vi "Instr_InitObject.vi"(8 "error in (no error)":errorcluster, 9 "Instrument Configuration":variant, 10 "Instrument address":refnum<visa-resource-name>, 11 "KE6517 in":refnum<class "KE6517.lvclass">) -> (0 "error out":errorcluster, 3 "KE6517 out":refnum<class "KE6517.lvclass">)   [LabVIEW 2018, in "KE6517.lvclass"]
uses:
  KE6517.lvclass
  InstrumentSetup.vi
  KE6517_CommandsGlobal.vi
  SupplyControl.lvclass
  InstrControl.lvclass
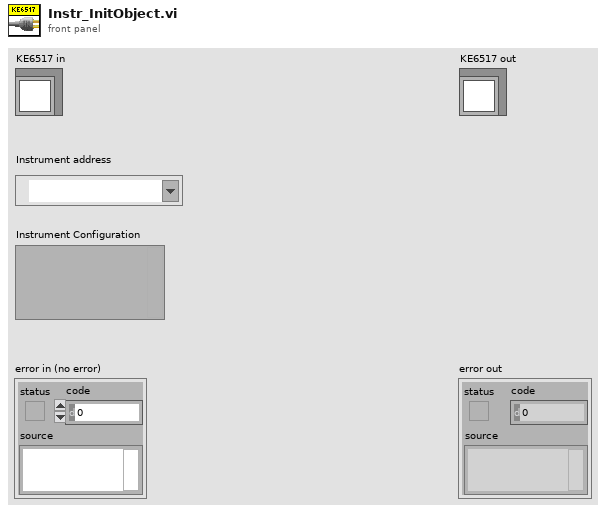
[diagram p1: front panel]
types:
  T1 = cluster{"Compliance [A]":sgl, "Voltage range (source)":enum16{"Auto", "200 V", "500 V", "1500 V", "3000 V"}, "Current range (measure)":enum16{"Auto", "1 nA", "10 nA", "100 nA", "1 uA", "10 uA", "100 uA", "1 mA", "2 mA", "20 mA", "120 mA"}, "KE2657A":refnum<class "KE2657A.lvclass">}
  T2 = cluster{"Instrument name":string, "Command \"Reset\"":string, "Command \"Initialise\"":string, "Command \"Arm\"":string, "Command \"SetVolts\"":string, "Command \"Compliance?\"":string, "Command \"Standby\"":string, "Command \"Read Current\"":string}
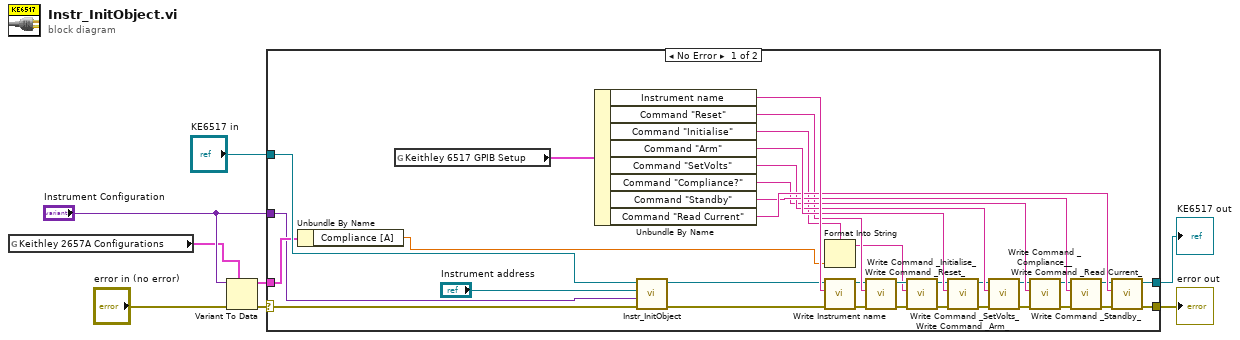
[diagram p0: block diagram]
diagram:
  n1 = global read "InstrumentSetup.vi" "Keithley 2657A Configurations"() -> (w2:T1)
  n2 = Variant To Data(error in="error in (no error)", type=w2, Variant="Instrument Configuration") -> (data=w1:T1, error out=w4:errorcluster)
  n3 = case shown="No Error" w4 {
    selector: w4 -> [w12 w44]
    tunnel: [w22 w44] -> w6
    tunnel: [w23 w43] -> w7
    tunnel: "KE6517 in" -> [w15 w43]
    tunnel: w1 -> [w10 _]
    tunnel: "Instrument Configuration" -> [w9 _]
    frame No Error {
      n4 = Unbundle By Name(w10) -> ("Compliance [A]"=w21:sgl)
      n5 = global read "KE6517_CommandsGlobal.vi" "Keithley 6517 GPIB Setup"() -> (w18:T2)
      n6 = Unbundle By Name(w18) -> ("Instrument name"=w42:string, "Command \"Reset\""=w36:string, "Command \"Initialise\""=w20:string, "Command \"Arm\""=w41:string, "Command \"SetVolts\""=w38:string, "Command \"Compliance?\""=w37:string, "Command \"Standby\""=w39:string, "Command \"Read Current\""=w40:string)
      n7 = call-parent "Instr_InitObject.vi"("error in (no error)"=w12, "Instrument Configuration"=w9, "Instrument address"="Instrument address", "SupplyControl in"=w15) -> ("error out"=w11:errorcluster, "SupplyControl out"=w14:refnum<class "KE6517.lvclass">)  [unwired: 6 in]
      n8 = Format Into String(format string=w20, w21) -> (resulting string=w19:string)  [unwired: 2 in, 1 out]
      n9 = call-dynamic "Write Instrument name.vi"("error in (no error)"=w11, "Instrument name"=w42, "InstControl in"=w14) -> ("error out"=w16:errorcluster, "InstControl out"=w17:refnum<class "KE6517.lvclass">)  [unwired: 7 in]
      n10 = call-dynamic "Write Command _Reset_.vi"("error in (no error)"=w16, "Command \"Reset\""=w36, "SupplyControl in"=w17) -> ("error out"=w29:errorcluster, "SupplyControl out"=w35:refnum<class "KE6517.lvclass">)  [unwired: 7 in]
      n11 = call-dynamic "Write Command _Initialise_.vi"("error in (no error)"=w29, "Command \"Initialise\""=w19, "SupplyControl in"=w35) -> ("error out"=w28:errorcluster, "SupplyControl out"=w34:refnum<class "KE6517.lvclass">)  [unwired: 7 in]
      n12 = call-dynamic "Write Command _Arm_.vi"("error in (no error)"=w28, "Command \"Arm\""=w41, "SupplyControl in"=w34) -> ("error out"=w27:errorcluster, "SupplyControl out"=w33:refnum<class "KE6517.lvclass">)  [unwired: 7 in]
      n13 = call-dynamic "Write Command _SetVolts_.vi"("error in (no error)"=w27, "Command \"SetVolts\""=w38, "SupplyControl in"=w33) -> ("error out"=w26:errorcluster, "SupplyControl out"=w32:refnum<class "KE6517.lvclass">)  [unwired: 7 in]
      n14 = call-dynamic "Write Command _Compliance__.vi"("error in (no error)"=w26, "Command \"Compliance?\""=w37, "SupplyControl in"=w32) -> ("error out"=w25:errorcluster, "SupplyControl out"=w31:refnum<class "KE6517.lvclass">)  [unwired: 7 in]
      n15 = call-dynamic "Write Command _Standby_.vi"("error in (no error)"=w25, "Command \"Standby\""=w39, "SupplyControl in"=w31) -> ("error out"=w24:errorcluster, "SupplyControl out"=w30:refnum<class "KE6517.lvclass">)  [unwired: 7 in]
      n16 = call-dynamic "Write Command _Read Current_.vi"("error in (no error)"=w24, "Command \"Read Current\""=w40, "SupplyControl in"=w30) -> ("error out"=w22:errorcluster, "SupplyControl out"=w23:refnum<class "KE6517.lvclass">)  [unwired: 7 in]
    }
    frame Error {
    }
  }
  "error out" <- w6
  "KE6517 out" <- w7
